vi "Find Best Cost.vi"(8 "error in (no error)":errorcluster, 10 "LRU Cache Size":i32, 11 "State in":refnum<class "State.lvclass">) -> (0 "error out":errorcluster, 3 "State out":refnum<class "State.lvclass">)   [LabVIEW 2019, in "23.lvlib" / "State.lvclass"]
uses:
  State.lvclass
  lv2019-LRU-Cache/LRU Cache/LRU Cache.lvclass
  lv2019-LRU-Cache/LRU Cache/LRU Cache.lvclass/LRU Cache.ctl
  lv2019-LRU-Cache/LRU DLL/LRU DLL.lvclass
  C:/Users/craig.walker/Documents/GitHub/lv2019-Doubly-Linked-List/Doubly Linked List/Doubly Linked List.lvclass
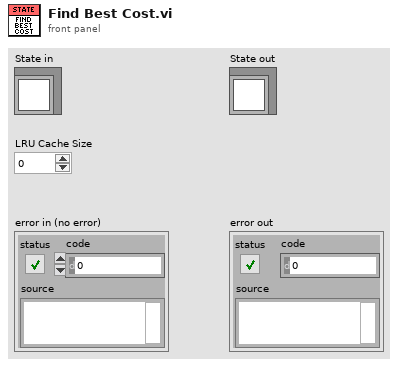
[diagram p1: front panel]
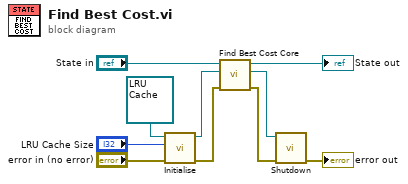
[diagram p0: block diagram]
diagram:
  n1 = call "Initialise.vi"("error in (no error)"="error in (no error)", "Maximum Size"="LRU Cache Size", "LRU Cache in"=refnum<class "LRU Cache.lvclass"> refnum) -> ("error out"=w7:errorcluster, "LRU Cache out"=w2:refnum<class "LRU Cache.lvclass">)  [unwired: 7 in]
  n2 = call "Find Best Cost Core.vi"("error in (no error)"=w7, "LRU Cache in"=w2, "State in"="State in") -> ("error out"=w9:errorcluster, "LRU Cache out"=w8:refnum<class "LRU Cache.lvclass">, "State out"=→"State out":refnum<class "State.lvclass">)  [unwired: 6 in]
  n3 = call "Shutdown.vi"("error in (no error)"=w9, "LRU Cache Queue in"=w8) -> ("error out"=→"error out":errorcluster)  [unwired: 9 in]
